vi "Vec2P3D.vi"(11 "Vec":dbl[](array[numeric])) -> (3 "P0":cluster{"X":dbl, "Y":dbl, "Z":dbl})   [LabVIEW 2014]
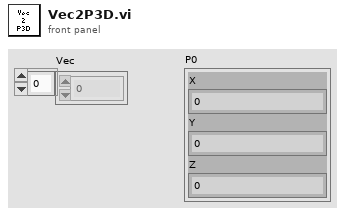
[diagram p1: front panel]
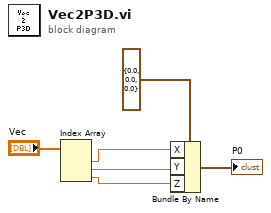
[diagram p0: block diagram]
diagram:
  n1 = Index Array(array="Vec") -> (element #1=w3:dbl, element #2=w2:dbl, element #3=w1:dbl)  [unwired: 3 in]
  n2 = Bundle By Name(cluster=cluster{"X":dbl, "Y":dbl, "Z":dbl} {"X"=0.0, "Y"=0.0, "Z"=0.0} ("P0"), "X"=w3, "Y"=w2, "Z"=w1) -> (→"P0":cluster{"X":dbl, "Y":dbl, "Z":dbl})
